vi "dispense off_n.vi"(8 "error in":errorcluster, 9 "dispense status in":bool, 10 "dispense":T1={"Vacuum Setting (0000)"=0, "Pressure"=20, "on delay (ms)"=0.5, "off delay (ms) "=0.5} {"Vacuum Setting (0000)" min=0 max=1000 step=1 format="%04.0f"}, 11 "Ultimus V2.lvclass":refnum<class "Ultimus V2.lvclass">) -> (0 "error out":errorcluster, 3 "Ultimus V2.lvclass 2":refnum<class "Ultimus V2.lvclass">)   [LabVIEW 2016]
uses:
  Classes/Controller/Dispenser/Ultimus V2 Folder/Ultimus V2.lvclass
panel:
  out "dispense status out":bool
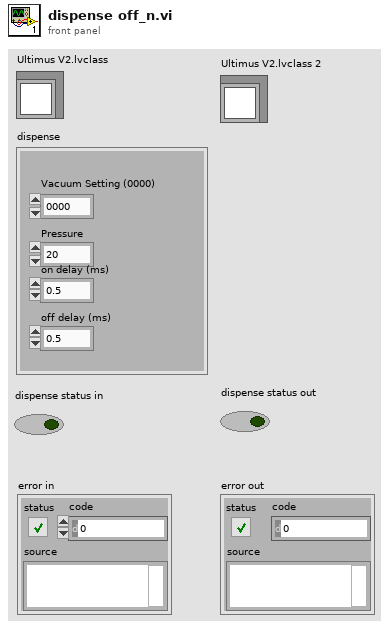
[diagram p1: front panel]
types:
  T1 = cluster{"Vacuum Setting (0000)":i64, "Pressure":i16, "on delay (ms)":dbl, "off delay (ms) ":dbl}
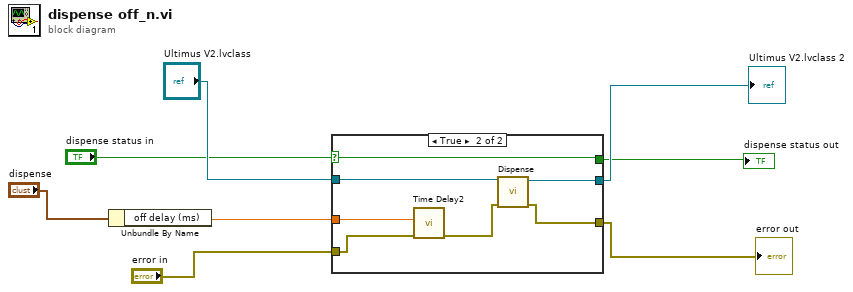
[diagram p0: block diagram]
diagram:
  n1 = Unbundle By Name("dispense") -> ("off delay (ms)"=w2:dbl)
  n2 = case shown="True" "dispense status in" {
    selector: "dispense status in" -> [w9 w12]
    tunnel: [w11 w18] -> w5
    tunnel: "Ultimus V2.lvclass" -> [w11 w17]
    tunnel: "error in" -> [w10 w14]
    tunnel: [w10 w16] -> w6
    tunnel: w2 -> [_ w13]
    tunnel: [w9 w12] -> w1
    frame False {
    }
    frame True {
      n3 = call "Time Delay2"("error in (no error)"=w14, "Delay Time (s)"=w13) -> ("error out"=w15:errorcluster)  [unwired: 9 in]
      n4 = call-dynamic "Dispense.vi"("error in (no error)"=w15, "Ultimus V in"=w17) -> ("error out"=w16:errorcluster, "Ultimus V out"=w18:refnum<class "Ultimus V2.lvclass">)  [unwired: 8 in]
    }
  }
  "Ultimus V2.lvclass 2" <- w5
  "error out" <- w6
  "dispense status out" <- w1
